vi "UI.vi"(10 "Numeric Control":dbl) -> ()   [LabVIEW 2015]
panel:
  in  "Stop Button":bool
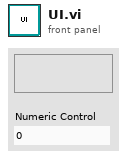
[diagram p1: front panel]
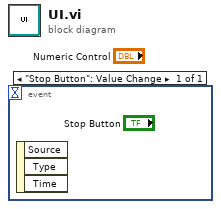
[diagram p0: block diagram]
diagram:
  n1 = event shown="[0] \"Stop Button\": Value Change" {
    selector: _ -> [_]
    dyn-events: _ -> [_]
    timeout: _ -> [_]
    event "Stop Button": Value Change {
      n2 = event-data() -> ()  [unwired: 1 in, 3 out]
    }
  }
